vi "nonlinear spring constant objective function.vi"(9 "output selector":T1, 10 "data":variant, 11 "X":dbl[](array[numeric])) -> (0 "error out":errorcluster, 1 "inequality constraint function values":dbl[](array[numeric]), 2 "equality constraint function values":dbl[](array[numeric]), 3 "objective function value":dbl)   [LabVIEW 2023]
doc: "Create the nonlinear spring constant objective function to be passed to the Constrained Nonlinear Optimization.vi."
uses:
  <vilib>/gmath/NumericalOptimization/cno_output select.ctl
  <vilib>/Simulation/Utility/Implementation/Shared/SIM Diagram Parameters.ctl
  <vilib>/Simulation/Implementation/Shared/SIM Continuous Solvers.ctl
  <vilib>/gmath/NI_Gmath.lvlib
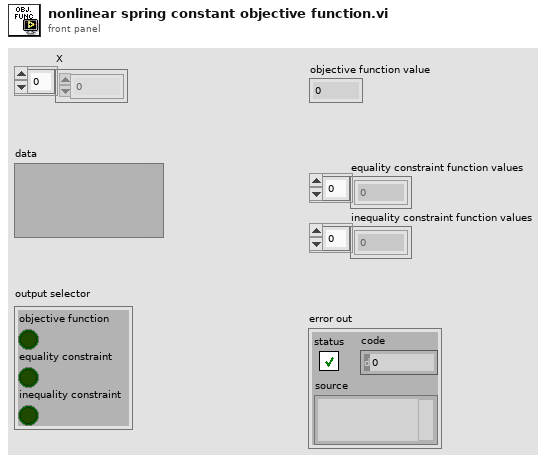
[diagram p1: front panel]
types:
  T1 = typedef "NI_Gmath.lvlib/cno_output select.ctl" = cluster{"objective function":bool, "equality constraint":bool, "inequality constraint":bool}
  T2 = typedef "SIM Continuous Solvers.ctl" = enum16{"Runge-Kutta 1 (Euler)", "Runge-Kutta 2", "Runge-Kutta 3", "Runge-Kutta 4", "Runge-Kutta 23 (variable)", "Runge-Kutta 45 (variable)", "BDF (variable)", "Adams-Moulton (variable)", "Rosenbrock (variable)", "Discrete States Only"}
  T3 = typedef "SIM Diagram Parameters.ctl" = cluster{"Initial Time":dbl, "Final Time":dbl, "Time Step":dbl, "Absolute Tolerance":dbl, "Relative Tolerance":dbl, "Continuous Solver":T2, "Discrete Time Step":dbl, "Minimum Time Step":dbl, "Maximum Time Step":dbl, "Initial Time Step":dbl}
  T4 = cluster{"outputs":dbl[][], "times":dbl[], "Initial conditions":dbl[], "simulation parameters":T3, "current simulation":refnum<vi>, "spring constant (initial guess)":refnum<vi>}
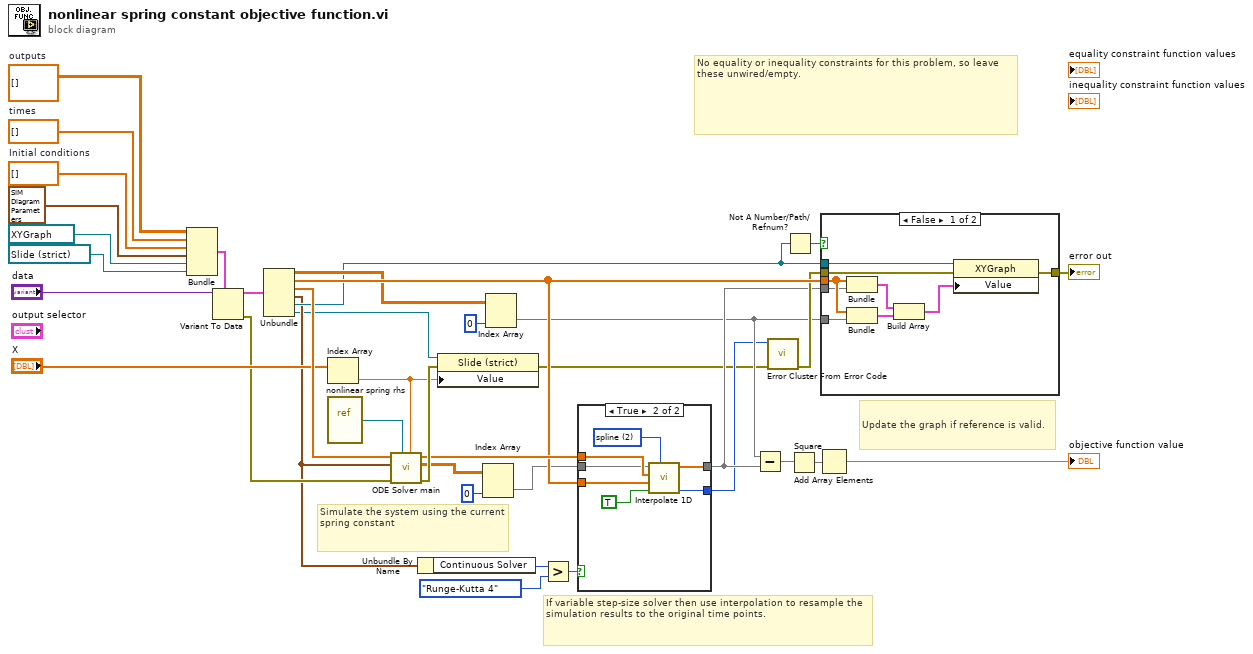
[diagram p0: block diagram]
diagram:
  w13 = dbl[] []  # Initial conditions
  w14 = dbl[] []  # times
  w15 = dbl[][] []  # outputs
  # "No equality or inequality constraints for this problem, so leave these unwired/empty."
  # "Update the graph if reference is valid."
  # "Simulate the system using the current spring constant"
  # "If variable step-size solver then use interpolation to resample the simulation results to the original time points."
  n1 = Bundle("outputs"=w15, "times"=w14, "Initial conditions"=w13, "simulation parameters"=T3 {"Initial Time"=0.0, "Final Time"=10.0, "Time Step"=0.1, "Absolute Tolerance"=0.001, "Relative Tolerance"=1e-07, "Continuous Solver"=enum."Runge-Kutta 45 (variable)", "Discrete Time Step"=1.0, "Minimum Time Step"=1e-08, "Maximum Time Step"=1.0, "Initial Time Step"=0.01}, "current simulation"=refnum<vi> refnum, "spring constant (initial guess)"=refnum<vi> refnum) -> (w11:T4)  [unwired: 1 in]
  n2 = Variant To Data(type=w11, Variant="data") -> (data=w36:T4, error out=w31:errorcluster)  [unwired: 1 in]
  n3 = Unbundle(w36) -> ("outputs"=w21:dbl[][], "times"=w28:dbl[], "Initial conditions"=w34:dbl[], "simulation parameters"=w9:T3, "current simulation"=w19:refnum<vi>, "spring constant (initial guess)"=w4:refnum<vi>)
  n4 = Index Array(array="X") -> (element=w3:dbl)  [unwired: 1 in]
  n5 = vi-ref "nonlinear spring rhs.vi"() -> (w35:refnum<vi>)
  n6 = call <vilib>:"ODE Solver main.vi"("data"=w3, "ODE F(X,t)"=w35, "error in (no error)"=w31, "simulation parameters"=w9, "x0"=w34) -> ("error out"=w38:errorcluster, "outputs"=w26:dbl[][], "times"=w32:dbl[])  [unwired: 4 in]
  n7 = Unbundle By Name(w9) -> ("Continuous Solver"=w8:T2)
  n8 = property class="Slide (strict)"(reference=w4, error in=w38, "Value"=w3) -> (error out=w1:errorcluster)  [unwired: 1 out]
  n9 = Index Array(array=w26, index (col)=0 ("disabled index (col)")) -> (element=w24:dbl[])  [unwired: 1 in]
  n10 = Index Array(array=w21, index (col)=0 ("index (row)")) -> (element=w20:dbl[])  [unwired: 1 in]
  n11 = Greater?(x=w8, y=SIM_Continuous_Solvers."Runge-Kutta 4") -> (0:w6:bool)
  n12 = case shown="True" w6 {
    tunnel: w32 -> [_ w46]
    tunnel: w28 -> [_ w45]
    tunnel: w24 -> [w39 w42]
    tunnel: [w39 w41] -> w22
    tunnel: [_ w40] -> w10
    frame False {
    }
    frame True {
      w43 = 2 items=["nearest", "linear", "spline", "cubic Hermite", "Lagrange"] ("method")
      n13 = call <vilib>:"Interpolate 1D.vi"("method"=w43, "X is monotonic"=TRUE, "xi"=w45, "X"=w46, "Y"=w42) -> ("error"=w40:i32, "yi"=w41:dbl[])  [unwired: 4 in, 1 out]
    }
  }
  n14 = Subtract(x=w20, y=w22) -> (x-y=w17:dbl[])
  n15 = call <vilib>:"Error Cluster From Error Code.vi"("error in (no error)"=w1, "error code (0)"=w10) -> ("error out"=w27:errorcluster)  [unwired: 7 in]
  n16 = Not A Number/Path/Refnum?(number/path/refnum=w19) -> (NaN/Path/Refnum?=w29:bool)
  n17 = Square(x=w17) -> (x^2=w18:dbl[])
  n18 = Add Array Elements(numeric array=w18) -> (sum=→"objective function value":dbl)
  n19 = case shown="False" w29 {
    tunnel: w19 -> [w55 _]
    tunnel: w22 -> [w47 _]
    tunnel: w28 -> [w52 _]
    tunnel: w27 -> [w54 w56]
    tunnel: [w53 w56] -> w30
    tunnel: w20 -> [w48 _]
    frame False {
      n20 = Bundle("times"=w52, "yi"=w47) -> (w51:cluster{"times":dbl[], "yi":dbl[]})  [unwired: 1 in]
      n21 = Bundle("times"=w52, "outputs"=w48) -> (w50:cluster{"times":dbl[], "outputs":dbl[]})  [unwired: 1 in]
      n22 = Build Array(w51, w50) -> (w49:cluster{"times":dbl[], "outputs":dbl[]}[])
      n23 = property class="XYGraph"(reference=w55, error in=w54, "Value"=w49) -> (error out=w53:errorcluster)  [unwired: 1 out]
    }
    frame True {
    }
  }
  "error out" <- w30
